vi "Temperature conversion.vi"(10 "Stop":bool, 11 "Celsius":dbl) -> (3 "Fahrenheit":dbl)   [LabVIEW 2014]
doc: "VI to convert C to F"
panel:
  # "Program to convert celsius to Fahrenheit"
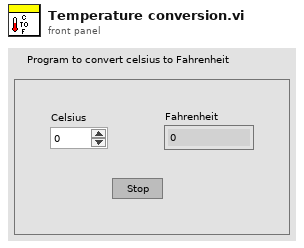
[diagram p1: front panel]
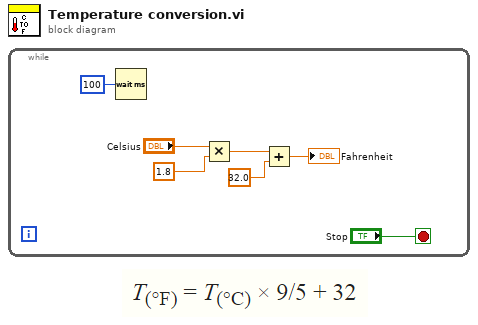
[diagram p0: block diagram]
diagram:
  n1 = while {
    stop <- "Stop" stop-if-true
    n2 = Wait (ms)(milliseconds to wait=u32 100) -> ()  [unwired: 1 out]
    n3 = Multiply(x="Celsius", y=1.8 ("Numeric")) -> (x*y=w2:dbl)
    n4 = Add(x=w2, y=32.0 ("Numeric")) -> (x+y=→"Fahrenheit":dbl)
  }
